vi "Initialize Modules Page.vi"(8 "error in (no error)":errorcluster, 10 "Modules Page Controls":T2, 11 "Routing and Faulting Ref in":T1 format="%.0x") -> (0 "error out":errorcluster, 3 "Routing and Faulting Ref out":T1 format="%.0x")   [LabVIEW 2017, in "Routing and Faulting System Explorer.lvlib"]
uses:
  Routing and Faulting System Explorer.lvlib
  Modules Page Controls.ctl
  <vilib>/NI Veristand/Custom Device API/Custom Device Item Ref.ctl
  Module Row.ctl
  Scripting/Routing and Faulting Scripting.lvlib
  <vilib>/NI Veristand/Custom Device API/Custom Device API.lvlib
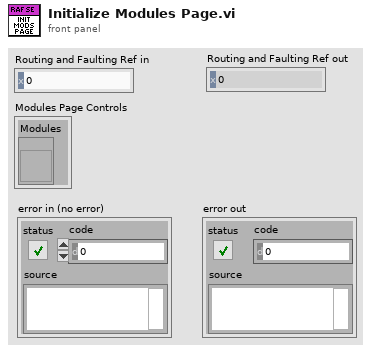
[diagram p1: front panel]
types:
  T1 = typedef "Custom Device API.lvlib/Custom Device Item Ref.ctl" = u64
  T2 = typedef "Routing and Faulting System Explorer.lvlib/Modules Page Controls.ctl" = cluster{"Modules":refnum<vi>}
  T3 = enum8{"Enabled", "Disabled", "Disabled and Grayed Out"}
  T4 = typedef "Routing and Faulting Shared.lvlib/Alias Mapping.ctl" = cluster{"Alias":string, "Endpoint":T5}
  T5 = typedef "Routing and Faulting Shared.lvlib/Alias Endpoint.ctl" = cluster{"Module Path":string, "Endpoint":string}
  T6 = typedef "Routing and Faulting Shared.lvlib/Channel States.ctl" = T7[]
  T7 = typedef "Routing and Faulting Shared.lvlib/Routing State.ctl" = cluster{"Name":string, "Description":string, "Value":i32, "Connection List":T8[]}
  T8 = typedef "Routing and Faulting Shared.lvlib/Connection.ctl" = cluster{"Module":string, "Source":string, "Destination":string}
  T9 = typedef "Routing and Faulting System Explorer.lvlib/Module Row.ctl" = cluster{"Module path":string, "Edit":bool, "Description":string}
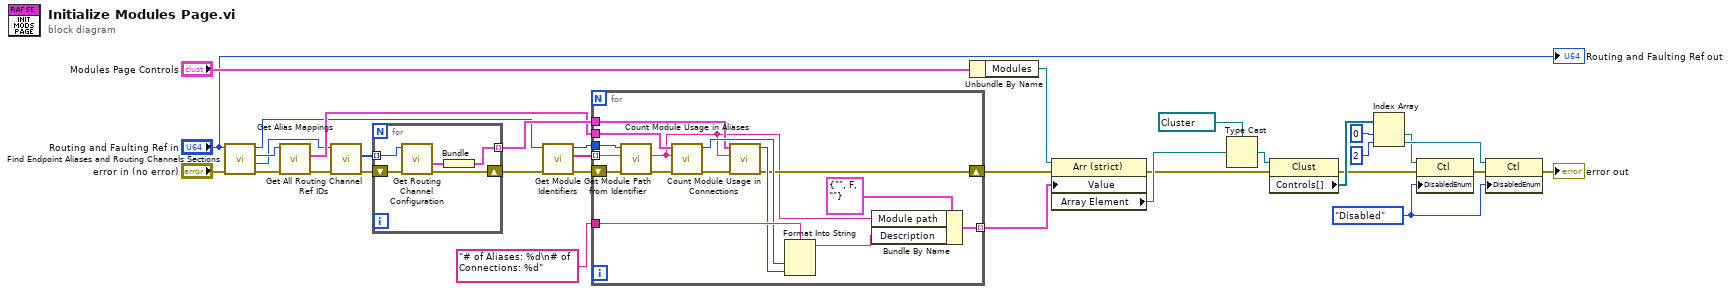
[diagram p0: block diagram]
diagram:
  w4 = T3."Disabled" ("Disabled")
  n1 = call "Find Endpoint Aliases and Routing Channels Sections.vi"("error in (no error)"="error in (no error)", "Routing and Faulting Custom Device Ref in"="Routing and Faulting Ref in") -> ("error out"=w12:errorcluster, "Routing Channels Ref"=w16:T1, "Endpoint Aliases Ref"=w17:T1, "Routing and Faulting Custom Device Ref out"=w9:T1)  [unwired: 6 in]
  n2 = call "Get Alias Mappings.vi"("error in (no error)"=w12, "Endpoint Aliases Ref in"=w17) -> ("error out"=w11:errorcluster, "Alias Mappings"=w18:T4[])  [unwired: 7 in, 1 out]
  n3 = call "Get All Routing Channel Ref IDs.vi"("error in (no error)"=w11, "Routing Channels Ref in"=w16) -> ("error out"=w19:errorcluster, "Channel Refs"=w20:T1[])  [unwired: 7 in, 1 out]
  n4 = for {
    tunnel: w20 -> [w37] mode=indexing
    shift-right: [w36] -> w10
    shift-left: w19 -> [w38]
    tunnel: [w34] -> w23 mode=indexing
    n5 = call "Get Routing Channel Configuration.vi"("error in (no error)"=w38, "Channel Ref in"=w37) -> ("error out"=w36:errorcluster, "State Configurations"=w35:T6)  [unwired: 4 in, 4 out]
    n6 = Bundle("State Configurations"=w35) -> (w34:cluster{"State Configurations":T6})  [unwired: 1 in]
  }
  n7 = call "Get Module Identifiers.vi"("error in (no error)"=w10, "Routing and Faulting Ref in"=w9) -> ("error out"=w13:errorcluster, "Module Identifiers"=w15:string[], "Routing and Faulting Ref out"=w14:T1)  [unwired: 7 in]
  n8 = for {
    shift-right: [w42] -> w8
    shift-left: w13 -> [w53]
    tunnel: w14 -> [w52]
    tunnel: w15 -> [w51] mode=indexing
    tunnel: w18 -> [w46]
    tunnel: "# of Aliases: %d\n# of Connections: %d" ("format string") -> [w49]
    tunnel: [w47] -> w22 mode=indexing
    tunnel: w23 -> [w41]
    n9 = call "Get Module Path from Identifier.vi"("error in (no error)"=w53, "Module identifier"=w51, "Routing and Faulting Ref in"=w52) -> ("error out"=w50:errorcluster, "Module path"=w40:string)  [unwired: 6 in, 1 out]
    n10 = call "Count Module Usage in Aliases.vi"("error in (no error)"=w50, "Module path"=w40, "Alias Mappings"=w46) -> ("error out"=w43:errorcluster, "Number of Usages"=w45:i32)  [unwired: 7 in]
    n11 = call "Count Module Usage in Connections.vi"("error in (no error)"=w43, "Module path"=w40, "All State Configurations"=w41) -> ("error out"=w42:errorcluster, "Number of Usages"=w44:i32)  [unwired: 7 in]
    n12 = Format Into String(format string=w49, w45, w44) -> (resulting string=w48:string)  [unwired: 2 in, 1 out]
    n13 = Bundle By Name(cluster=T9 {"Module path"="", "Edit"=FALSE, "Description"=""} ("Modules"), "Module path"=w40, "Description"=w48) -> (w47:T9)
  }
  n14 = Unbundle By Name("Modules Page Controls") -> ("Modules"=w33:refnum<vi>)
  n15 = property class="Arr (strict)"(reference=w33, error in=w8, "Value"=w22) -> (error out=w7:errorcluster, "Array Element"=w24:refnum<vi>)  [unwired: 1 out]
  n16 = Type Cast(type=refnum<vi> refnum ("Array Element"), x=w24) -> (*(type *) &x=w29:refnum<vi>)
  n17 = property class="Clust"(reference=w29, error in=w7) -> (error out=w6:errorcluster, "Controls[]"=w28:refnum<vi>[])  [unwired: 1 out]
  n18 = Index Array(array=w28, index #1=0 ("index"), index #2=2 ("index")) -> (element #1=w30:refnum<vi>, element #2=w31:refnum<vi>)
  n19 = property class="Ctl"(reference=w30, error in=w6, "DisabledEnum"=w4) -> (error out=w5:errorcluster)  [unwired: 1 out]
  n20 = property class="Ctl"(reference=w31, error in=w5, "DisabledEnum"=w4) -> (error out=→"error out":errorcluster)  [unwired: 1 out]
  "Routing and Faulting Ref out" <- "Routing and Faulting Ref in"
